vi "Configuration Database FGV.vi"(8 "error in":errorcluster, 9 "Record to add/replace/query":T1, 10 "UDL file for Client SQL Database":path, 11 "Action":T4=enum."Query Timing Data") -> (0 "error out":errorcluster, 2 "Wash Duration":dbl, 3 "Records":T1[](array[typedef]))   [LabVIEW 2018, in "Controller.lvlib"]
uses:
  Controller.lvlib
  Common/ctl/Wash Step.ctl
  Common/Common.lvlib
  Common/ctl/Station.ctl
  ctl/Database Record.ctl
  ctl/Database Action.ctl
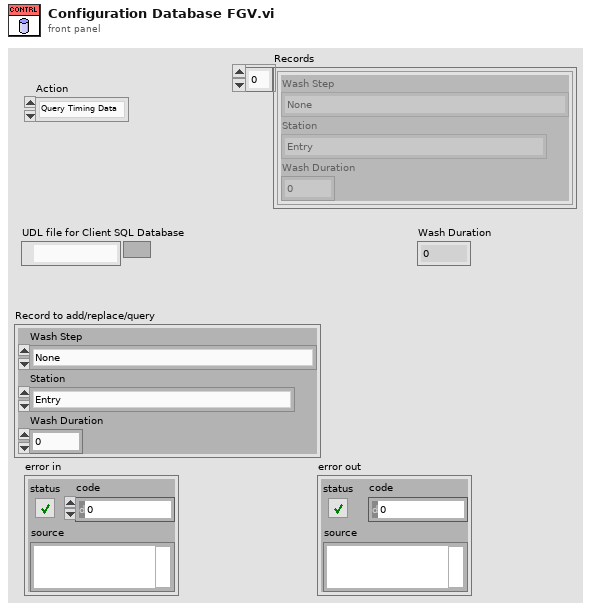
[diagram p1: front panel]
types:
  T1 = typedef "Controller.lvlib/Database Record.ctl" = cluster{"Wash Step":T2, "Station":T3, "Wash Duration":dbl}
  T2 = typedef "Common.lvlib/Wash Step.ctl" = enum16{"None", "Under Body Wash", "Bug Remover", "Pre-Soak", "High Pressure Wash (default)", "Low Pressure Wax", "Spot Free Rinse", "Tire Shine Foam", "Air Dry"}
  T3 = typedef "Common.lvlib/Station.ctl" = enum16{"Entry", "Station 1", "Station 2", "Station 3", "Exit"}
  T4 = typedef "Controller.lvlib/Database Action.ctl" = enum16{"Read Records (init)", "Get", "Query Timing Data", "Insert New Data record", "Update Data Record"}
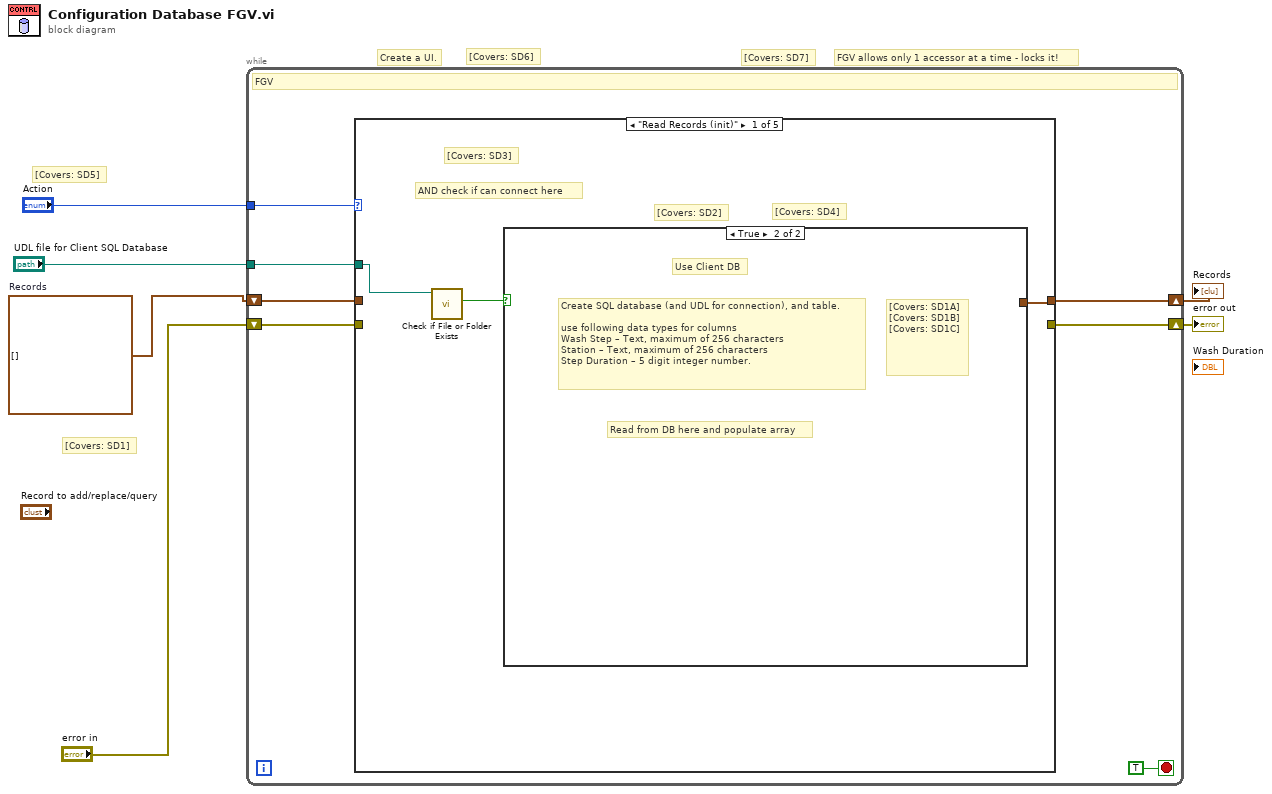
[diagram p0: block diagram]
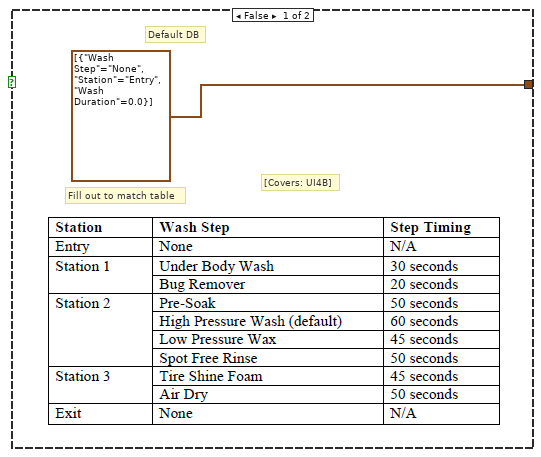
[diagram p2: hidden frame]
diagram:
  w2 = T1[] []  # Records
  # "[Covers: SD5]"
  # "[Covers: SD6]"
  # "FGV allows only 1 accessor at a time - locks it!"
  # "[Covers: SD7]"
  # "Create a UI."
  # "[Covers: SD1]"
  n1 = while {
    tunnel: "Action" -> [w13]
    shift-right: [w10] -> w5
    shift-left: "error in" -> [w9]
    shift-right: [w11] -> w1
    shift-left: w2 -> [w8]
    tunnel: "UDL file for Client SQL Database" -> [w7]
    stop <- TRUE stop-if-true
    # "FGV"
    n2 = case shown="\"Read Records (init)\"" w13 {
      tunnel: [w14 w19 _ _ _] -> w11
      tunnel: [_ w18 _ _ _] -> w10
      tunnel: w9 -> [_ w18 _ _ _]
      tunnel: w8 -> [_ w19 _ _ _]
      tunnel: w7 -> [w16 _ _ _ _]
      frame "Read Records (init)" {
        # "[Covers: SD4]"
        # "[Covers: SD2]"
        # "AND check if can connect here"
        # "[Covers: SD3]"
        n3 = call <vilib>:"Check if File or Folder Exists.vi"("path"=w16) -> ("file or folder exists?"=w15:bool)  [unwired: 8 in, 2 out]
        n4 = case shown="True" w15 {
          tunnel: [T1[] [{"Wash Step"=enum."None", "Station"=enum."Entry", "Wash Duration"=0.0}] ("Records") _] -> w14
          frame False {
            # "Default DB"
            # "[Covers: UI4B]"
            # "Fill out to match table"
          }
          frame True {
            # "[Covers: SD1A]\n[Covers: SD1B]\n[Covers: SD1C]"
            # "Create SQL database (and UDL for connection), and table.\n\nuse following data types for columns\nWash Step – Text, maximum of 256 characters\nStation – Text, maximum of 256 characters\nStep Duration – 5 digit integer number."
            # "Read from DB here and populate array"
            # "Use Client DB"
          }
        }
      }
      frame "Get", Default {
      }
      frame "Query Timing Data" {
      }
      frame "Insert New Data record" {
        # "Complete this"
      }
      frame "Update Data Record" {
        # "Complete this"
      }
    }
  }
  "error out" <- w5
  "Records" <- w1
